vi "Global_Map Data.vi"() -> ()   [LabVIEW 2015]
panel:
  in  "Hot Spots":i32[][](array[numeric])
  in  "MoveTrack":i32[][](array[numeric])
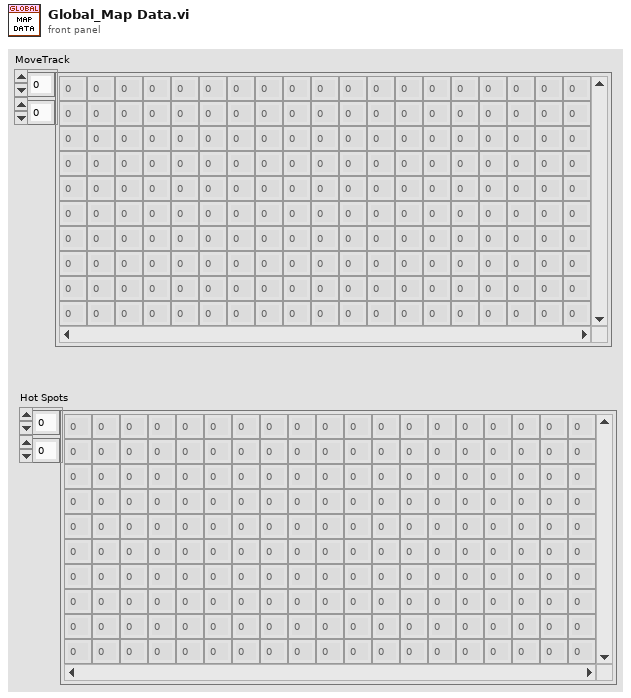
[diagram p1: front panel]
diagram:
